vi "Write Severity.vi"(8 "error in":errorcluster, 10 "severity":T1, 11 "Has Alarm in":refnum<class "Has Alarm.lvclass">) -> (0 "error out":errorcluster, 3 "Has Alarm out":refnum<class "Has Alarm.lvclass">)   [LabVIEW 2020, in "PV Access.lvlib" / "PV Data.lvlib" / "Has Alarm.lvclass"]
uses:
  Has Alarm.lvclass
  Alarm Severity.ctl
  PV Data.lvlib
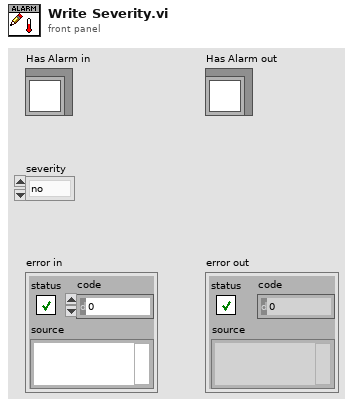
[diagram p1: front panel]
types:
  T1 = typedef "PV Access.lvlib/PV Data.lvlib/Alarm Severity.ctl" = enum32{"no", "minor", "major", "record", "invalid", "undefined"}
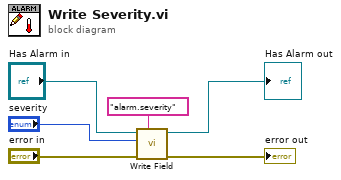
[diagram p0: block diagram]
diagram:
  n1 = call-dynamic "Write Field.vi"("field"="alarm.severity", "error in (no error)"="error in", "value"="severity", "Base Interface in"="Has Alarm in") -> ("error out"=→"error out":errorcluster, "Base Interface out"=→"Has Alarm out":refnum<class "Has Alarm.lvclass">)  [unwired: 6 in]
